vi "Waveform Chart_single point.vi"() -> ()   [LabVIEW 2020]
panel:
  out "Waveform Chart":dbl(graph)
  in  "Go":bool
  in  "stop":bool
  in  "Clear Chart":bool
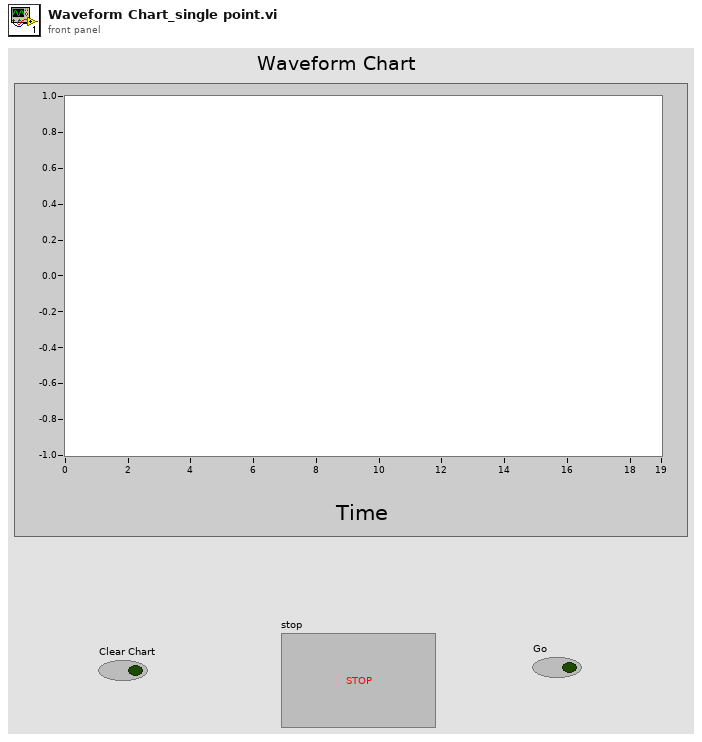
[diagram p1: front panel]
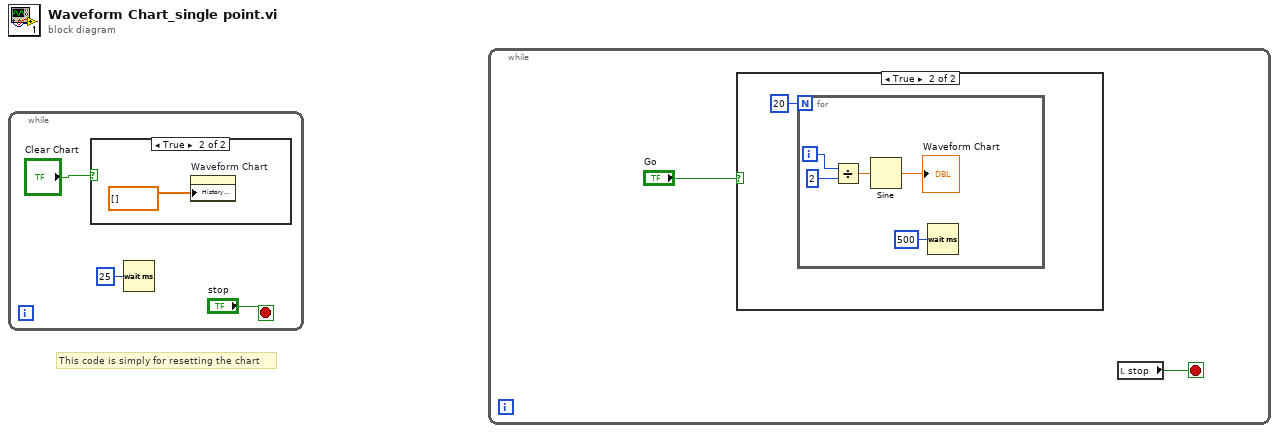
[diagram p0: block diagram]
diagram:
  # "This code is simply for resetting the chart"
  n1 = while {
    stop <- "stop" stop-if-true
    n2 = case shown="True" "Clear Chart" {
      frame False {
      }
      frame True {
        n3 = property on="Waveform Chart" class="WFChart (strict)"("History Data"=dbl[] []) -> ()  [unwired: 2 in, 2 out]
      }
    }
    n4 = Wait (ms)(milliseconds to wait=u32 25) -> ()  [unwired: 1 out]
  }
  n5 = while {
    stop <- w6 stop-if-true
    n6 = case shown="True" "Go" {
      frame False {
      }
      frame True {
        n7 = for {
          N: 20 -> [_]
          i -> [w10]
          n8 = Divide(x=w10, y=2) -> (x/y=w8:dbl)
          n9 = Sine(x=w8) -> (sin(x)=→"Waveform Chart":dbl)
          n10 = Wait (ms)(milliseconds to wait=u32 500) -> ()  [unwired: 1 out]
        }
      }
    }
    n11 = local read "stop"() -> (w6:bool)
  }
